vi "ChromaPowerSupply.vi"() -> ()   [LabVIEW 2018, in "Visualization.lvlib" / "VisualizeAcPwr.lvclass"]
doc: "This VI listens for any measurement data associated with the provided PluginName and displays it to the user for analysis. The display is only suitable for data coming from the RoomAlert Plugin."
uses:
  VisualizeAcPwr.lvclass
  VisualizeBase/VisualizeBase_class/SubVIs/VisualizationOptions.ctl
  <vilib>/Utility/miscctls.llb/LVRectTypeDef.ctl
  Loop Parameters.ctl
  AcPwr/AcPwrShared/clMeasurmentData.ctl
  AcPwr/AcPwrPlugins/AcPwrBaseClass/TypeDefs/SetParameterInputs.ctl
  AcPwr/AcPwrPlugins/ChromaPowerSupplyClass/TypeDefs/Device(s)Settings.ctl
  AcPwr/AcPwrPlugins/ChromaPowerSupplyClass/TypeDefs/Measurements.ctl
  <vilib>/event_ctls.llb/usereventprio.ctl
  VisualizeBase/VisualizeBase_class/Requests/VisUserEventType.ctl
  <vilib>/Utility/error.llb/Error Cluster From Error Code.vi
  <vilib>/ErrorRing/Error Ring.xnode
  <userlib>/NIST/NISTErrorLib/NISTErrorLib.lvlib
  VisualizeBase/VisualizeBase_class/VisualizeBase.lvclass
  TestClass/Test.lvclass
  Sensor/VisualizeSensor.lvclass
  StatusAndLog/VisualizeStatus.lvclass
  AcPwr/AcPwrShared/AcPwrShared.lvlib
  AcPwr/AcPwrPlugins/ChromaPowerSupplyClass/ChromaPowerSupply.lvclass
  AcPwr/AcPwrModule/AcPwrModule.lvlib
  AcPwr/AcPwrPlugins/AcPwrPlugins.lvlib
  AcPwr/AcPwrPlugins/AcPwrBaseClass/AcPwrBase.lvclass
panel:
  out "Writetime":u32 caption="Sample Write Time(ms)"
  out "ExitHelperLoops?":bool
  in  "Display":enum16{"Raw Data", "Voltage Vs Current"}(ring)
  in  "btnPause":bool
  out "VisualizationProperties":T1={"PauseAtStartup"=TRUE, "LogData"=FALSE, "LaunchInSubPanel"=TRUE, "FPMonitor"=0, "FPWindowBounds"={"Left"=0, "Top"=0, "Right"=0, "Bottom"=0}, "MonitorBounds"={"Left"=0, "Top"=0, "Right"=0, "Bottom"=0}, "MeasIndices"=[]}
  in  "INIFilePath":path
  in  "ModuleID":i32
  in  "Log Data":bool=TRUE
  in  "btnStop":bool
  in  "btnReset":bool
  in  "btnClearTest":bool
  in  "btnStopModule":bool
  out "XY Graph":cluster{dbl[], dbl[]}(graph)
  out "Chart":waveform(dbl)[](graph)=[{"t0"=timestamp(3657200531.6397257 s since 1904-01-01), "dt"=1.0, "Y"=[46.19]}, {"t0"=timestamp(3657200531.6397257 s since 1904-01-01), "dt"=1.0, "Y"=[2.0]}, {"t0"=timestamp(3657200531.6397257 s since 1904-01-01), "dt"=1.0, "Y"=[60.0]}]
  in  "Current":bool
  in  "Voltage":bool
  in  "Current (A)":dbl
  in  "Voltage (V)":dbl
  in  "btnStopParameterLoop":bool
  in  "btnRunParamLoop":bool
  in  "Loop Parameters":T3={"Parameter"=enum."Voltage", "Start Value"=5.0, "Increment"=1.0, "Interval (s)"=3.0, "# Iterations"=6, "End Value"=10.0} {"# Iterations" min=1; "Increment" format="%#.4f"}
  out "ErrorArray":errorcluster[](array[cluster])
  out "Incorrect DataType?":bool
  out "String Results":string
  in  "PluginName":string="Sensor.RoomAlert1"
  # "Set Parameter"
  # "Parameter Looping"
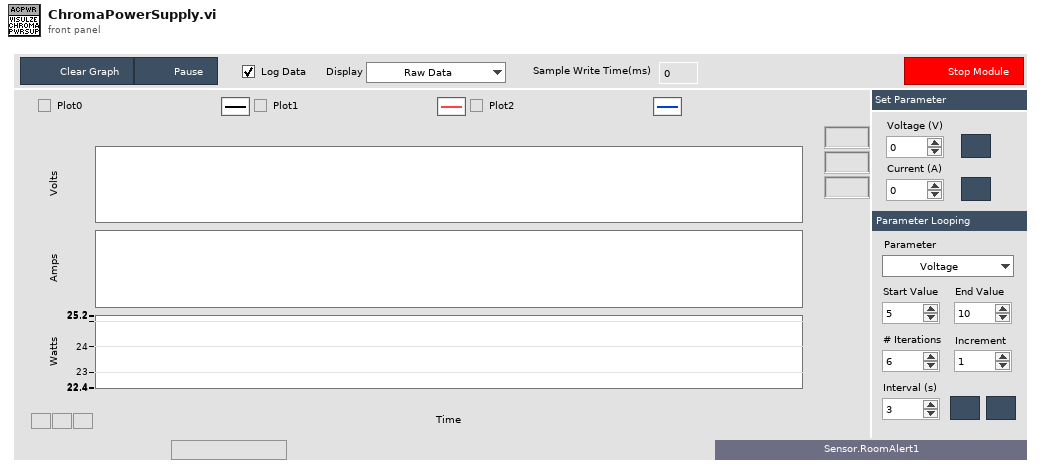
[diagram p1: front panel]
types:
  T1 = typedef "Visualization.lvlib/VisualizeBase.lvclass/VisualizationOptions.ctl" = cluster{"PauseAtStartup":bool, "LogData":bool, "LaunchInSubPanel":bool, "FPMonitor":u16, "FPWindowBounds":T2, "MonitorBounds":cluster{"Left":i16, "Top":i16, "Right":i16, "Bottom":i16}, "MeasIndices":i32[]}
  T2 = typedef "LVRectTypeDef.ctl" = cluster{"Left":i16, "Top":i16, "Right":i16, "Bottom":i16}
  T3 = typedef "Loop Parameters.ctl" = cluster{"Parameter":enum16{"Voltage", "Current", "Power", "Resistance"}, "Start Value":dbl, "Increment":dbl, "Interval (s)":dbl, "# Iterations":u32, "End Value":dbl}
  T4 = enum16{"open", "open or create", "create or replace", "create", "open (read-only)"}
  T5 = typedef "Visualization.lvlib/VisualizeBase.lvclass/VisRequestEvents.ctl" = cluster{"StopRequest":refnum<user-event>, "ResetRequest":refnum<user-event>, "FP Pop In or Out":refnum<user-event>}
  T6 = typedef "AcPwrShared.lvlib/AcPwrBroadcastEvents.ctl" = cluster{"DidInit":refnum<user-event>, "StatusUpdate":refnum<user-event>, "ErrorReport":refnum<user-event>, "DidStop":refnum<user-event>, "PathToINI":refnum<user-event>, "Measurements":refnum<user-event>, "LoadConfigFile":refnum<user-event>, "GetSettings":refnum<user-event>, "SetSettings":refnum<user-event>, "GetType&ID":refnum<user-event>, "GotSettings":refnum<user-event>, "GotSettingsLV":refnum<user-event>, "ParameterSet":refnum<user-event>}
  T7 = typedef "Visualization.lvlib/VisualizeBase.lvclass/VisFrmWrkBroadcastEvents.ctl" = cluster{"StatusUpdate":refnum<user-event>, "DidStop":refnum<user-event>, "NewModuleLoaded":refnum<user-event>, "StopVisualization":refnum<user-event>}
  T8 = typedef "AcPwrShared.lvlib/clMeasurmentData.ctl" = cluster{"MeasName":string, "XML Data":string, "WaveformData":waveform(dbl)[]}
  T9 = typedef "AcPwrPlugins.lvlib/AcPwrBase.lvclass/SetParameterInputs.ctl" = cluster{"Type":string, "Parameter":string, "Phase":i32, "Value":dbl, "Command":string, "Time Stamp":timestamp}
  T10 = typedef "AcPwrPlugins.lvlib/ChromaPowerSupply.lvclass/Device(s)Settings.ctl" = cluster{"Phases":cluster{"Handle":string, "Instrument Options":string, "id query (T)":bool, "reset device (T)":bool, "Timing":cluster{"TimingOn":enum16{""}, "Hours":u32, "Minutes":u32, "Seconds":dbl, "CutoffVoltage":dbl}, "Connected":bool, "Output Mode":enum16{"Voltage (DC)", "Current (DC)"}, "Voltage":dbl, "Current":dbl, "High Voltage Limit":dbl, "High Current Limit":dbl, "Power Protect":dbl, "Current Protect":dbl, "Voltage Protect":dbl, "Low Current Limit":dbl, "Low Voltage Limit":dbl, "Current Slew Rate":dbl, "Voltage Slew Rate":dbl, "Current Slew Infinite?":bool}[], "MeasName":string}
  T11 = typedef "AcPwrPlugins.lvlib/ChromaPowerSupply.lvclass/Measurements.ctl" = cluster{"Handle":string, "Name":string, "Enabled":bool, "Measurement Value":dbl, "btnMeasFetch":bool, "ProtectionStatusString":string, "Measurement Type":enum16{"Voltage", "Current", "Power"}}[]
  T12 = cluster{"Device Settings":T10, "Measurements":T11}
  T13 = typedef "Visualization.lvlib/VisualizeBase.lvclass/VisUserEventType.ctl" = cluster{"BusIndex":i8, "Data":variant}
  T14 = typedef "usereventprio.ctl" = enum32{"high priority", "normal priority"}
  T15 = cluster{"Handle":string, "Instrument Options":string, "id query (T)":bool, "reset device (T)":bool, "Timing":cluster{"TimingOn":enum16{""}, "Hours":u32, "Minutes":u32, "Seconds":dbl, "CutoffVoltage":dbl}, "Connected":bool, "Output Mode":enum16{"Voltage (DC)", "Current (DC)"}, "Voltage":dbl, "Current":dbl, "High Voltage Limit":dbl, "High Current Limit":dbl, "Power Protect":dbl, "Current Protect":dbl, "Voltage Protect":dbl, "Low Current Limit":dbl, "Low Voltage Limit":dbl, "Current Slew Rate":dbl, "Voltage Slew Rate":dbl, "Current Slew Infinite?":bool}[]
  T16 = cluster{"Handle":string, "Instrument Options":string, "id query (T)":bool, "reset device (T)":bool, "Timing":cluster{"TimingOn":enum16{""}, "Hours":u32, "Minutes":u32, "Seconds":dbl, "CutoffVoltage":dbl}, "Connected":bool, "Output Mode":enum16{"Voltage (DC)", "Current (DC)"}, "Voltage":dbl, "Current":dbl, "High Voltage Limit":dbl, "High Current Limit":dbl, "Power Protect":dbl, "Current Protect":dbl, "Voltage Protect":dbl, "Low Current Limit":dbl, "Low Voltage Limit":dbl, "Current Slew Rate":dbl, "Voltage Slew Rate":dbl, "Current Slew Infinite?":bool}
  T17 = typedef "sizeaction.ctl" = enum32{"Minimized", "Maximized", "Resized"}
  T18 = enum16{"Voltage", "Current", "Power", "Resistance"}
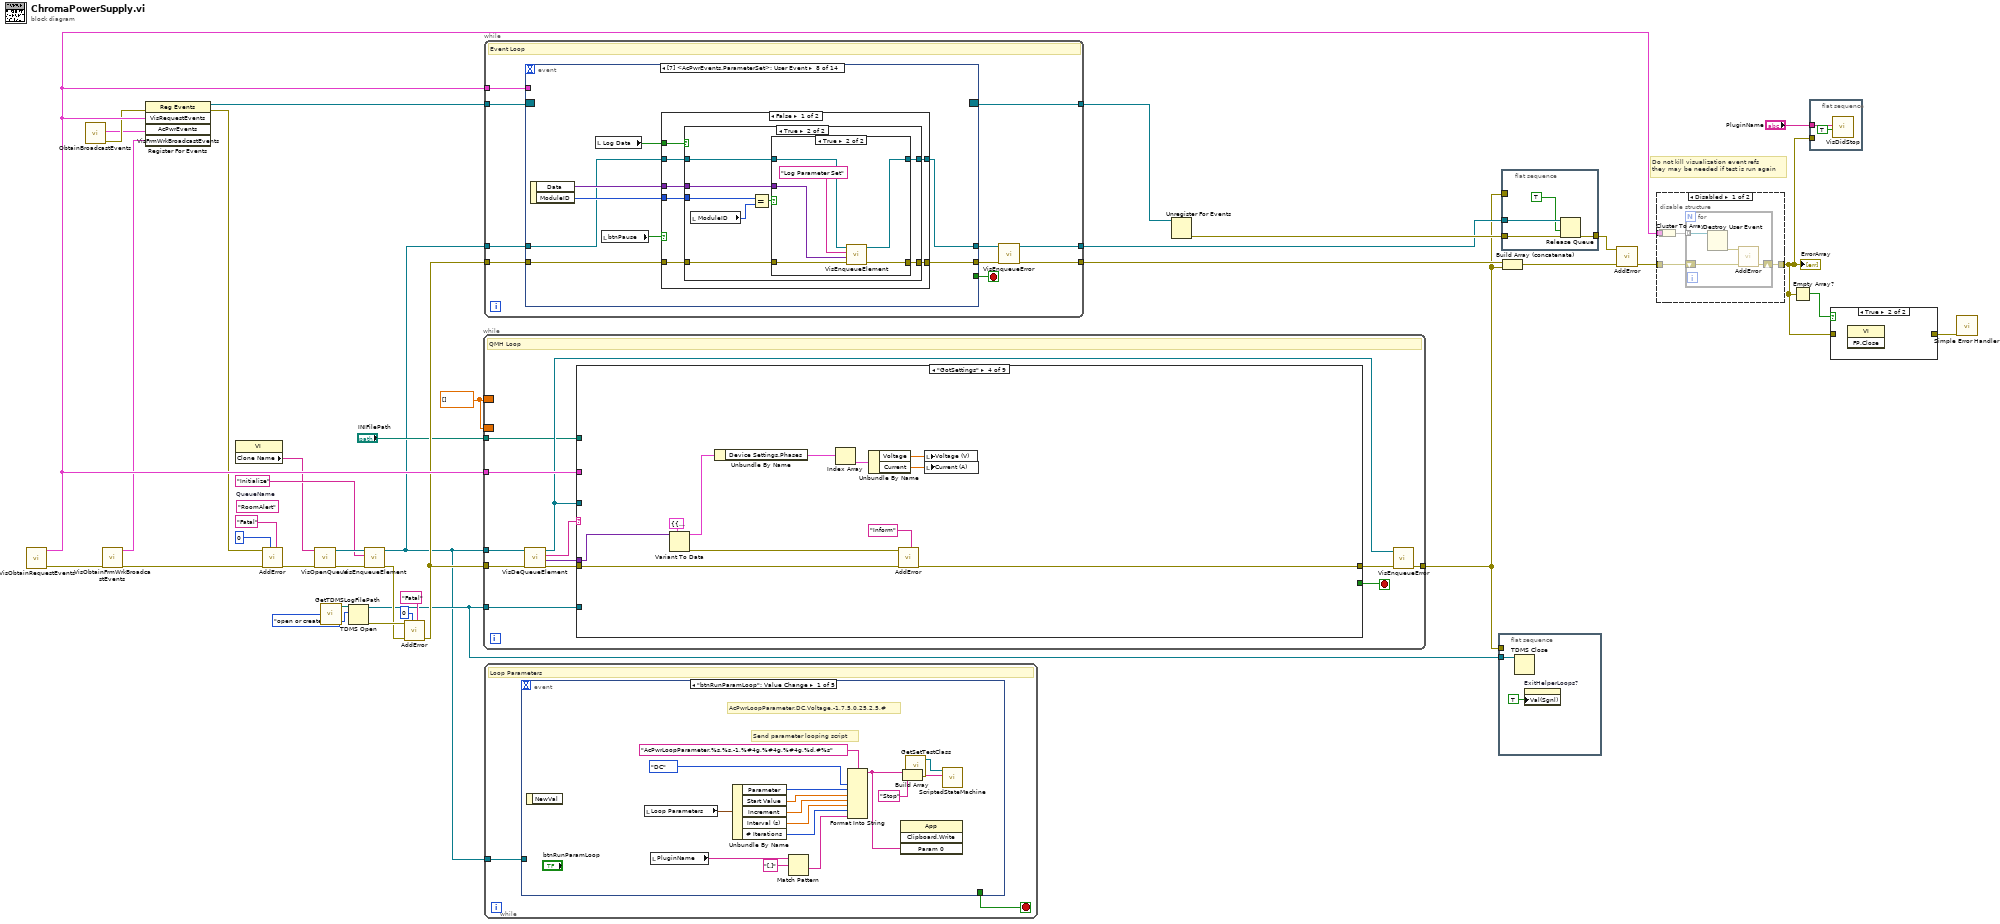
[diagram p0: block diagram]
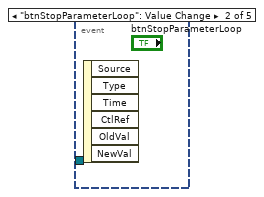
[diagram p2: hidden frame]
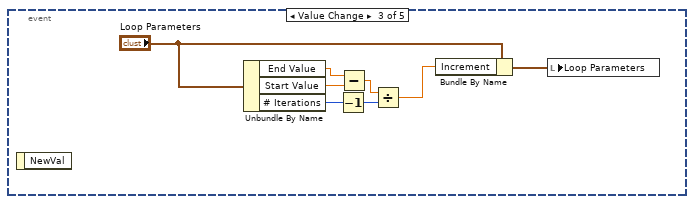
[diagram p3: hidden frame]
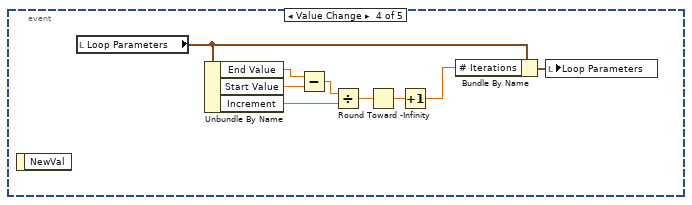
[diagram p4: hidden frame]
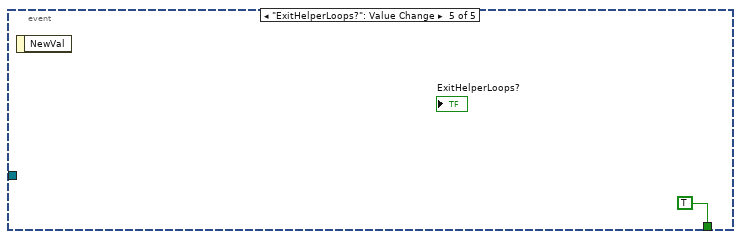
[diagram p5: hidden frame]
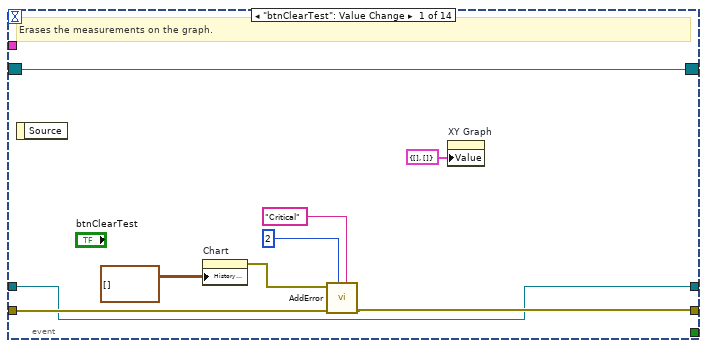
[diagram p7: hidden frame]
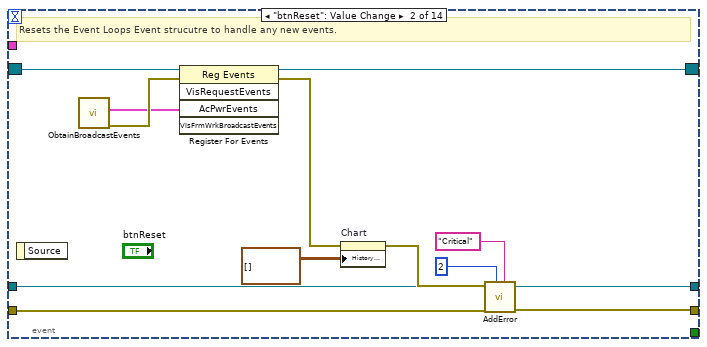
[diagram p8: hidden frame]
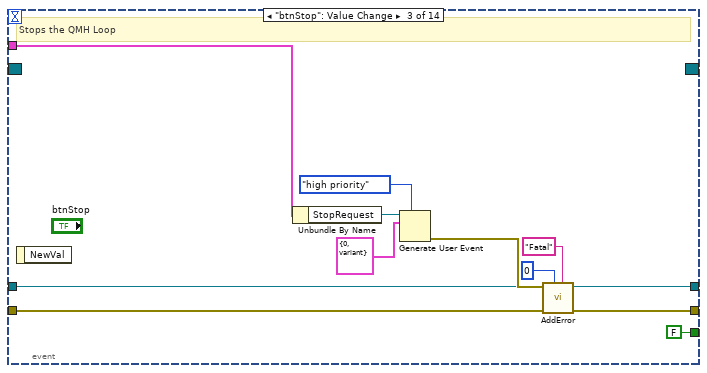
[diagram p9: hidden frame]
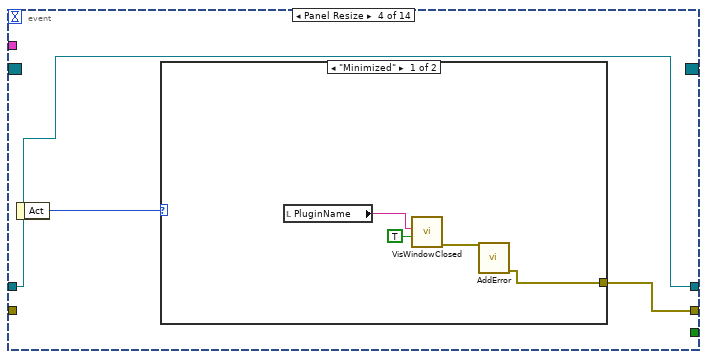
[diagram p10: hidden frame]
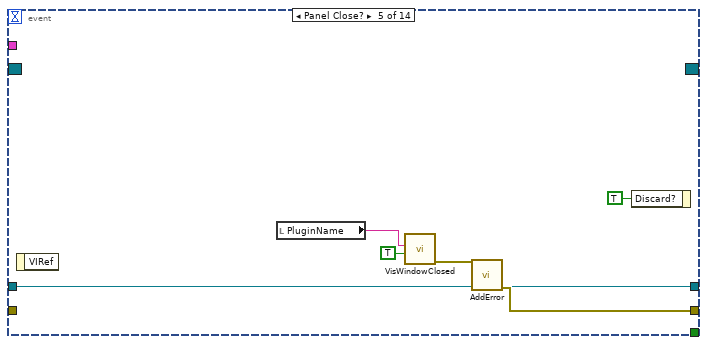
[diagram p12: hidden frame]
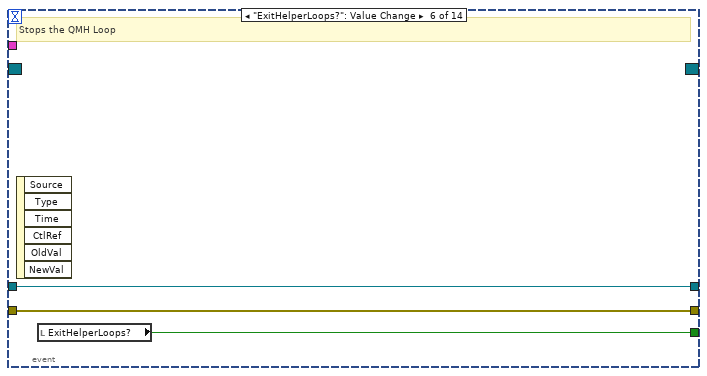
[diagram p13: hidden frame]
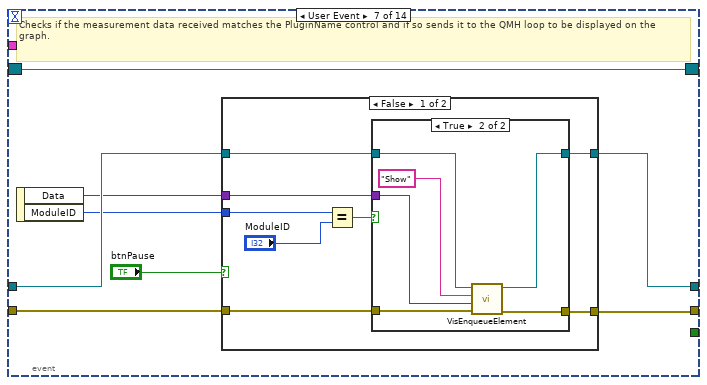
[diagram p14: hidden frame]
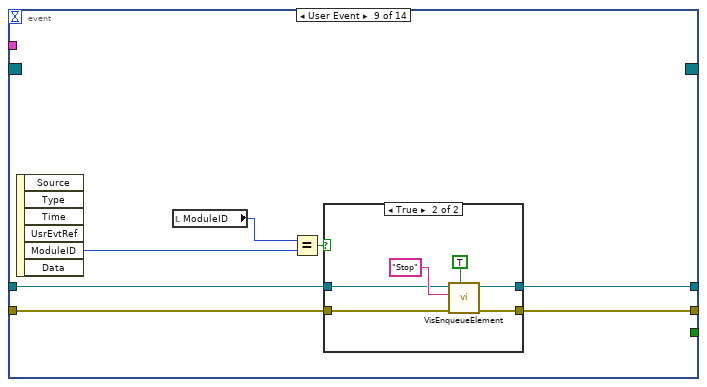
[diagram p20: hidden frame]
diagram:
  w1 = dbl[] []
  (unwired) "RoomAlert"  # QueueName
  # "Do not kill visualization event refs\nthey may be needed if test is run again"
  n1 = call "VisObtainRequestEvents.vi"() -> ("Error"=w29:errorcluster[], "VisRequestEvents"=w31:T5)  [unwired: 10 in]
  n2 = call "ObtainBroadcastEvents.vi"() -> ("error out"=w25:errorcluster, "AcPwrEvents"=w18:T6)  [unwired: 10 in]
  n3 = call "VisObtainFrmWrkBroadcastEvents.vi"("Error"=w29) -> ("Error"=w4:errorcluster[], "VisFrmWrkBroadcastEvents"=w3:T7)  [unwired: 9 in]
  n4 = register-events(error in=w25, w31, w18, w3) -> (reference out=w38:refnum<event-registration>, error out=w28:errorcluster)  [unwired: 1 in]
  n5 = property class="VI"() -> ("Clone Name"=w17:string)  [unwired: 2 in, 2 out]
  n6 = call <userlib>:"AddError.vi"("Severity"="Fatal", "Priority"=u8 0, "ErrorArray In"=w4, "error in (no error)"=w28) -> ("ErrorArray Out"=w24:errorcluster[])  [unwired: 6 in, 1 out]
  n7 = call "VisOpenQueue.vi"("Error Array In"=w24, "QueueName"=w17) -> ("Error Array Out"=w22:errorcluster[], "queue out"=w23:refnum<queue>)  [unwired: 8 in]
  n8 = call "GetTDMSLogFilePath.vi"() -> ("TDMS Log File Path"=w16:path)  [unwired: 11 in]
  n9 = TDMS Open(10:T4."open or create" ("operation (0:open)"), 11:w16) -> (0:w13:errorcluster, 3:w9:refnum<k34>)  [unwired: 5 in]
  n10 = call "VisEnqueueElement.vi"("Error Array In"=w22, "Message"="Initialize", "queue in"=w23) -> ("Error Array Out"=w12:errorcluster[], "queue out"=w2:refnum<queue>)  [unwired: 7 in]
  n11 = call <userlib>:"AddError.vi"("Severity"="Fatal", "Priority"=u8 0, "ErrorArray In"=w12, "error in (no error)"=w13) -> ("ErrorArray Out"=w11:errorcluster[])  [unwired: 6 in, 1 out]
  n12 = while {
    tunnel: w11 -> [w44]
    tunnel: [w47] -> w8
    tunnel: w2 -> [w43]
    tunnel: w31 -> [w49]
    tunnel: w9 -> [w40]
    tunnel: "INIFilePath" -> [w39]
    border: w1 -> [_]
    border: w1 -> [_]
    stop <- w50 stop-if-true
    # "QMH Loop"
    n13 = call "VisDeQueueElement.vi"("Error Array In"=w44, "Queue In"=w43) -> ("Error Array Out"=w42:errorcluster[], "Data"=w45:variant, "Message"=w46:string, "Queue Out"=w41:refnum<queue>)  [unwired: 6 in]
    n14 = case shown="\"GotSettings\"" w46 {
      selector: w46 -> [_ _ _ _ w174 _ _ _ _]
      tunnel: w45 -> [_ w72 w139 w164 _ w193 _ _ w235]
      tunnel: w42 -> [w61 w73 _ w162 w172 _ w222 _ w230]
      tunnel: [w54 w74 _ w161 w171 w183 w221 _ w232] -> w48
      tunnel: [_ _ _ _ _ w189 TRUE _ _] -> w50
      tunnel: w49 -> [_ _ _ _ _ w188 _ _ _]
      tunnel: w41 -> [_ _ _ _ _ w187 _ _ _]
      tunnel: w40 -> [_ w71 w138 _ _ _ _ _ _]
      tunnel: w39 -> [w60 _ _ _ _ _ w223 _ _]
      frame "Initialize" {
        n15 = property on="Chart" class="WFChart (strict)"("History Data"=waveform(dbl)[][] []) -> ()  [unwired: 2 in, 2 out]
        n16 = property on="XY Graph" class="XYGraph (strict)"("Value"=cluster{dbl[], dbl[]} {[], []} ("XY Graph")) -> ()  [unwired: 2 in, 2 out]
        n17 = call "ApplyVisOptions.vi"("INIFilePath"=w60) -> ("error out"=w64:errorcluster, "VisualizationProperties"=→"VisualizationProperties":T1)  [unwired: 9 in]
        n18 = call <userlib>:"AddError.vi"("Severity"="Inform", "ErrorArray In"=w61, "error in (no error)"=w64) -> ("ErrorArray Out"=w62:errorcluster[])  [unwired: 7 in, 1 out]
        n19 = property on="Display" class="Enum (strict)"("Val(Sgnl)"="Display") -> ()  [unwired: 2 in, 2 out]
        n20 = local read "ModuleID"() -> (w51:i32)
        n21 = call "GetSettingsRequestLV.vi"("SettingsToGet"=variant, "ModuleID"=w51) -> ("Error Out"=w53:errorcluster)  [unwired: 9 in]
        n22 = call <userlib>:"AddError.vi"("Severity"="Inform", "ErrorArray In"=w62, "error in (no error)"=w53) -> ("ErrorArray Out"=w54:errorcluster[])  [unwired: 7 in, 1 out]
      }
      frame "Show" {
        n23 = flat-sequence {
          tunnel: w71 -> [w76]
          tunnel: w72 -> [w77]
          tunnel: w73 -> [w78]
          tunnel: [w78] -> w70
          tunnel: [w77] -> w69
          tunnel: [w76] -> w68
          tunnel: [w75] -> w67
          tunnel: w70 -> [w92]
          tunnel: w69 -> [w91]
          tunnel: w68 -> [w86]
          tunnel: w67 -> [w79]
          tunnel: [w93] -> w66
          tunnel: [w79] -> w65
          tunnel: [w136] -> w74
          tunnel: w66 -> [w136]
          tunnel: w65 -> [w134]
          frame #0 {
            n24 = Tick Count (ms)() -> (millisecond timer value=w75:u32)
          }
          frame #1 {
            w88 = u32[] [0, 1, 2]  # PlotYAxis
            # "0=Left Axis and 1=Right Axis"
            n25 = Variant To Data(type=T8 {"MeasName"="", "XML Data"="", "WaveformData"=[]} ("MeasurmentDataCluster"), Variant=w91) -> (data=w89:T8, error out=w90:errorcluster)  [unwired: 1 in]
            n26 = control-ref of="Chart"() -> (w80:refnum<vi>)
            n27 = Unbundle By Name(w89) -> ("WaveformData"=w81:waveform(dbl)[])
            n28 = call "RetrieveAcPwrMeasurementData.vi"("WaveformChartReference"=w80, "PlotYScale"=w88, "WaveformArrayIn"=w81, "error in (no error)"=w90) -> ("WaveformArrayOut"=w83:waveform(dbl)[], "OutputString(Chroma)"=w85:string, "Incorrect DataType?"=w84:bool, "error out"=w87:errorcluster)  [unwired: 7 in, 1 out]
            n29 = case shown="False" w84 {
              selector: w84 -> [w107 _]
              tunnel: [w116 w132] -> w93
              tunnel: w92 -> [w115 w132]
              tunnel: w87 -> [w112 _]
              tunnel: w86 -> [w109 _]
              tunnel: w85 -> [w108 _]
              tunnel: w83 -> [w95 _]
              frame False {
                n30 = Array Size(array=w95) -> (size(s)=w94:i32)
                n31 = Index Array(array=w95, index #1=1 ("index"), index #2=0 ("index")) -> (element #1=w106:waveform(dbl), element #2=w105:waveform(dbl))
                n32 = property on="Chart" class="WFChart (strict)"("LegNumRows"=w94) -> ()  [unwired: 2 in, 2 out]
                n33 = Unbundle By Name(w106) -> ("Y"=w104:dbl[])
                n34 = Unbundle By Name(w105) -> ("Y"=w101:dbl[])
                n35 = feedback #1() -> (w103:dbl[])
                n36 = Build Array (concatenate)(w103, w104) -> (w98:dbl[])
                n37 = feedback-in #1(w98) -> ()
                n38 = feedback #2() -> (w102:dbl[])
                n39 = Build Array (concatenate)(w102, w101) -> (w97:dbl[])
                n40 = feedback-in #2(w97) -> ()
                n41 = Bundle(w98, w97) -> (→"XY Graph":cluster{dbl[], dbl[]})  [unwired: 1 in]
                n42 = case shown="True" "Log Data" {
                  tunnel: w112 -> [w117 w130]
                  tunnel: [w117 w131] -> w111
                  tunnel: w95 -> [_ w129]
                  tunnel: w109 -> [_ w124]
                  frame False {
                  }
                  frame True {
                    n43 = call "PrepareWaveformDataForTDMS.vi"("error in (no error)"=w130, "WaveformArray in"=w129) -> ("error out"=w128:errorcluster, "Measurement Data"=w126:dbl[][], "Channel Names"=w127:string[], "TimeStamp"=w119:timestamp)  [unwired: 6 in]
                    n44 = local read "PluginName"() -> (w122:string)
                    n45 = Build Array(w119) -> (w118:timestamp[])
                    n46 = TDMS Write(0:w124, 5:w122, 7:"TimeStamp" ("PluginName"), 9:w118, 11:w128) -> (4:w123:refnum<k34>, 6:w121:string, 15:w125:errorcluster)  [unwired: 1 in, 1 out]
                    n47 = TDMS Write(0:w123, 5:w121, 7:w127, 9:w126, 11:w125) -> (15:w131:errorcluster)  [unwired: 1 in, 3 out]
                  }
                }
                n48 = call <userlib>:"AddError.vi"("Severity"="Fatal" ("String"), "Priority"=u8 0, "ErrorArray In"=w115, "error in (no error)"=w111) -> ("ErrorArray Out"=w116:errorcluster[])  [unwired: 6 in, 1 out]
                "String Results" <- w108
                "Incorrect DataType?" <- w107
                "Chart" <- w95
              }
              frame True {
              }
            }
          }
          frame #2 {
            n49 = Tick Count (ms)() -> (millisecond timer value=w135:u32)
            n50 = Subtract(x=w135, y=w134) -> (x-y=→"Writetime":u32)
          }
        }
      }
      frame "Log Parameter Set" {
        n51 = Variant To Data(type=T9 {"Type"="", "Parameter"="", "Phase"=0, "Value"=0.0, "Command"="", "Time Stamp"=timestamp(0 s since 1904-01-01)}, Variant=w139) -> (data=w151:T9, error out=w140:errorcluster)  [unwired: 1 in]
        n52 = Unbundle By Name(w151) -> ("Type"=w150:string, "Parameter"=w149:string, "Phase"=w148:i32, "Time Stamp"=w144:timestamp, "Value"=w142:dbl)
        n53 = local read "PluginName"() -> (w137:string)
        n54 = Format Into String(format string="Set-%s_%s_Phase_%d", w150, w149, w148) -> (resulting string=w143:string)  [unwired: 2 in, 1 out]
        n55 = Concatenate Strings(w143, "_TimeStamp" ("string")) -> (w145:string)
        n56 = Build Array(w144) -> (w152:timestamp[])
        n57 = Build Array(w142) -> (w141:dbl[])
        n58 = TDMS Write(0:w138, 5:w137, 7:w145, 9:w152, 11:w140) -> (4:w154:refnum<k34>, 6:w153:string, 15:w155:errorcluster)  [unwired: 1 in, 1 out]
        n59 = TDMS Write(0:w154, 5:w153, 7:w143, 9:w141, 11:w155) -> ()  [unwired: 1 in, 4 out]
      }
      frame "GotSettings" {
        n60 = Variant To Data(type=T12 {"Device Settings"={"Phases"=[], "MeasName"=""}, "Measurements"=[]} ("output cluster"), Variant=w164) -> (data=w165:T12, error out=w160:errorcluster)  [unwired: 1 in]
        n61 = Unbundle By Name(w165) -> ("Device Settings.Phases"=w166:T15)
        n62 = Index Array(array=w166) -> (element=w167:T16)  [unwired: 1 in]
        n63 = Unbundle By Name(w167) -> ("Voltage"=w158:dbl, "Current"=w157:dbl)
        n64 = call <userlib>:"AddError.vi"("Severity"="Inform", "ErrorArray In"=w162, "error in (no error)"=w160) -> ("ErrorArray Out"=w161:errorcluster[])  [unwired: 7 in, 1 out]
        n65 = local write "Voltage (V)"(w158) -> ()
        n66 = local write "Current (A)"(w157) -> ()
      }
      frame Default {
        n67 = xnode "Error Ring"("parameter 0"=w174) -> ("error out"=w173:errorcluster)
        n68 = call <userlib>:"AddError.vi"("Severity"="Inform" ("String"), "Priority"=u8 5, "ErrorArray In"=w172, "error in (no error)"=w173) -> ("ErrorArray Out"=w171:errorcluster[], "error out"=w170:errorcluster)  [unwired: 6 in]
        n69 = call <vilib>:"Clear Errors.vi"("error in (no error)"=w170) -> ()  [unwired: 5 in, 2 out]
      }
      frame "Error" {
        n70 = Variant To Data(type=errorcluster[] [], Variant=w193) -> (data=w191:errorcluster[], error out=w182:errorcluster)  [unwired: 1 in]
        n71 = call <userlib>:"ParseErrors.vi"("ErrorArray"=w191) -> ("ErrorArray"=w190:errorcluster[])  [unwired: 8 in, 2 out]
        n72 = for {
          tunnel: w190 -> [w204] mode=indexing
          tunnel: [w198] -> w184 mode=concatenating
          tunnel: [w196] -> w189
          tunnel: w188 -> [w195]
          tunnel: w187 -> [w194]
          stop <- w196 stop-if-true
          n73 = call <userlib>:"GeneralHandler.vi"("error in (no error)"=w204) -> ("Severity"=w197:string, "Stop"=w201:bool, "Abort"=w202:bool, "Continue"=w203:bool)  [unwired: 6 in, 1 out]
          n74 = Build Array(w203, w202, w201) -> (w200:bool[])
          n75 = Boolean Array To Number(Boolean array=w200) -> (number=w199:u32)
          n76 = case shown="1" w199 {
            tunnel: [_ _ w209 w218] -> w198
            tunnel: w197 -> [_ _ _ w211]
            tunnel: [_ _ _ w213] -> w196
            tunnel: w195 -> [_ _ _ w212]
            tunnel: w194 -> [_ _ w205 _]
            frame 0, Default {
              # "No Dialog"
            }
            frame 1 {
              # "Continue"
            }
            frame 2 {
              # "Abort, Flush Queue"
              n77 = Flush Queue(queue=w205) -> (error out=w208:errorcluster)  [unwired: 1 in, 2 out]
              n78 = call <userlib>:"AddError.vi"("Severity"="Critical" ("String"), "Priority"=u8 1, "error in (no error)"=w208) -> ("ErrorArray Out"=w209:errorcluster[])  [unwired: 7 in, 1 out]
            }
            frame 4 {
              # "Stop"
              n79 = Unbundle By Name(w212) -> ("StopRequest"=w219:refnum<user-event>)
              n80 = Equal?(x=w211, y="Fatal" ("x")) -> (x = y?=w213:bool)
              n81 = Generate User Event(priority (normal)=usereventprio."high priority", user event=w219, event data cluster=T13 {"BusIndex"=0, "Data"=variant} ("event data")) -> (error out=w217:errorcluster)  [unwired: 1 in, 1 out]
              n82 = call <userlib>:"AddError.vi"("error in (no error)"=w217) -> ("ErrorArray Out"=w218:errorcluster[], "error out"=w214:errorcluster)  [unwired: 9 in]
              n83 = call <vilib>:"Clear Errors.vi"("error in (no error)"=w214) -> ()  [unwired: 5 in, 2 out]
            }
          }
        }
        n84 = call <userlib>:"AddError.vi"("Severity"="Critical", "Priority"=u8 2, "ErrorArray In"=w184, "error in (no error)"=w182) -> ("ErrorArray Out"=w183:errorcluster[])  [unwired: 6 in, 1 out]
      }
      frame "Stop" {
        n85 = local read "VisualizationProperties"() -> (w220:T1)
        n86 = call "WriteVisOptionsToINIFile.vi"("Visualization Options"=w220, "INIFilePath"=w223) -> ("error out"=w224:errorcluster)  [unwired: 8 in, 1 out]
        n87 = call <userlib>:"AddError.vi"("Severity"="Inform", "ErrorArray In"=w222, "error in (no error)"=w224) -> ("ErrorArray Out"=w221:errorcluster[])  [unwired: 7 in, 1 out]
      }
      frame "- ---AcPwr Module Specific Commands----" {
      }
      frame "Set Parameter" {
        n88 = Variant To Data(type="", Variant=w235) -> (data=w233:string, error out=w231:errorcluster)  [unwired: 1 in]
        n89 = call <userlib>:"AddError.vi"("Severity"="Inform", "Priority"=u8 0, "ErrorArray In"=w230, "error in (no error)"=w231) -> ("ErrorArray Out"=w227:errorcluster[])  [unwired: 6 in, 1 out]
        n90 = local read "PluginName"() -> (w243:string)
        n91 = case shown="\"False\", Default" w233 {
          tunnel: "Voltage (V)" -> [_ w254 _]
          tunnel: "Current (A)" -> [_ _ w255]
          tunnel: [_ w254 w255] -> w245
          tunnel: [TRUE _ _] -> w242
          frame "False", Default {
          }
          frame "Voltage" {
          }
          frame "Current" {
          }
        }
        n92 = Match Pattern(string=w243, regular expression="[.]") -> (after substring=w244:string)  [unwired: 1 in, 3 out]
        n93 = Format Into String(format string="AcPwrSetParameter,%s,%s,-1,%.4f,#%s", enum16{"AC", "DC"}."DC" ("input 1"), w233, w245, w244) -> (resulting string=w241:string)  [unwired: 2 in, 1 out]
        n94 = case shown="False" w242 {
          tunnel: w241 -> [w250 _]
          tunnel: [w248 w252] -> w232
          tunnel: w227 -> [w246 w252]
          frame False {
            n95 = call "GetSetTestClass.vi"() -> ("Test.lvclass"=w251:refnum<class "Test.lvclass">)  [unwired: 11 in]
            n96 = Build Array(w250, "Stop" ("element")) -> (w249:string[])
            n97 = call "ScriptedStateMachine.vi"("ErrorArray 2"=w246, "script"=w249, "Test.lvclass 2"=w251) -> ("ErrorArray"=w248:errorcluster[])  [unwired: 6 in, 2 out]
          }
          frame True {
          }
        }
      }
    }
    n98 = call "VisEnqueueError.vi"("Error Array In"=w48, "Queue in"=w41) -> ("Error Array Out"=w47:errorcluster[])  [unwired: 8 in, 1 out]
  }
  n99 = while {
    tunnel: w38 -> [w265]
    tunnel: [w259] -> w36
    tunnel: [w263] -> w37
    tunnel: w31 -> [w262]
    tunnel: w11 -> [w261]
    tunnel: w2 -> [w260]
    tunnel: [w256] -> w20
    stop <- w264 stop-if-true
    # "Event Loop"
    n100 = event shown="[7] <AcPwrEvents.ParameterSet>: User Event" {
      selector: w265 -> [w268 w286 _ _ _ _ w317 _ _ _ _ _ _ _]
      dyn-events: [w268 w285 _ _ _ _ w317 _ _ _ _ _ _ _] -> w263
      timeout: _ -> [_ _ _ _ _ _ _ _ _ _ _ _ _ _]
      tunnel: [_ _ FALSE ("Priority? (F)") _ _ w311 _ _ _ _ _ _ _ _] -> w264
      tunnel: [w271 w283 w290 w299 w306 w312 w319 w340 w378 _ w400 w408 w419 w429] -> w258
      tunnel: w262 -> [_ _ w289 _ _ _ _ _ _ _ _ _ _ _]
      tunnel: w261 -> [w272 w284 w297 _ _ w312 w320 w342 w377 _ _ w406 _ w428]
      tunnel: w260 -> [w266 w276 w287 w298 w305 w313 w321 w343 w380 w390 w398 w405 w418 w431]
      tunnel: [w266 w276 w287 w298 w305 w313 w318 w341 w379 w390 w399 w407 w418 w430] -> w257
      event "btnClearTest": Value Change {
        # "Erases the measurements on the graph."
        n101 = event-data() -> ()  [unwired: 1 in, 1 out]
        n102 = property on="Chart" class="WFChart (strict)"("History Data"=waveform(dbl)[][] []) -> (error out=w270:errorcluster)  [unwired: 2 in, 1 out]
        n103 = call <userlib>:"AddError.vi"("Severity"="Critical", "Priority"=u8 2, "ErrorArray In"=w272, "error in (no error)"=w270) -> ("ErrorArray Out"=w271:errorcluster[])  [unwired: 6 in, 1 out]
        n104 = property on="XY Graph" class="XYGraph (strict)"("Value"=cluster{dbl[], dbl[]} {[], []} ("XY Graph")) -> ()  [unwired: 2 in, 2 out]
      }
      event "btnReset": Value Change {
        # "Resets the Event Loops Event strucutre to handle any new events."
        n105 = event-data() -> ()  [unwired: 1 in, 1 out]
        n106 = call "ObtainBroadcastEvents.vi"() -> ("error out"=w277:errorcluster, "AcPwrEvents"=w275:T6)  [unwired: 10 in]
        n107 = register-events(reference=w286, error in=w277, w275) -> (reference out=w285:refnum<event-registration>, error out=w279:errorcluster)  [unwired: 2 in]
        n108 = property on="Chart" class="WFChart (strict)"(error in=w279, "History Data"=waveform(dbl)[][] []) -> (error out=w278:errorcluster)  [unwired: 1 in, 1 out]
        n109 = call <userlib>:"AddError.vi"("Severity"="Critical", "Priority"=u8 2, "ErrorArray In"=w284, "error in (no error)"=w278) -> ("ErrorArray Out"=w283:errorcluster[])  [unwired: 6 in, 1 out]
      }
      event "btnStop": Value Change {
        # "Stops the QMH Loop"
        n110 = event-data() -> ()  [unwired: 1 in, 1 out]
        n111 = Unbundle By Name(w289) -> ("StopRequest"=w295:refnum<user-event>)
        n112 = Generate User Event(priority (normal)=usereventprio."high priority", user event=w295, event data cluster=T13 {"BusIndex"=0, "Data"=variant} ("event data")) -> (error out=w296:errorcluster)  [unwired: 1 in, 1 out]
        n113 = call <userlib>:"AddError.vi"("Severity"="Fatal" ("String"), "Priority"=u8 0, "ErrorArray In"=w297, "error in (no error)"=w296) -> ("ErrorArray Out"=w290:errorcluster[])  [unwired: 6 in, 1 out]
      }
      event Panel Resize {
        n114 = event-data() -> ("Act"=w300:T17)  [unwired: 1 in]
        n115 = case shown="\"Minimized\"" w300 {
          tunnel: [w301 _] -> w299
          frame "Minimized" {
            n116 = local read "PluginName"() -> (w303:string)
            n117 = call "VisWindowClosed.vi"("Window Closed?"=TRUE ("Window Minimized or Clozed?"), "Module Name"=w303) -> ("error out"=w304:errorcluster)  [unwired: 9 in]
            n118 = call <userlib>:"AddError.vi"("error in (no error)"=w304) -> ("ErrorArray Out"=w301:errorcluster[])  [unwired: 9 in, 1 out]
          }
          frame "Maximized", Default {
          }
        }
      }
      event Panel Close? {
        n119 = event-data() -> ()  [unwired: 1 in, 1 out]
        n120 = local read "PluginName"() -> (w307:string)
        n121 = call "VisWindowClosed.vi"("Window Closed?"=TRUE ("Window Minimized or Clozed?"), "Module Name"=w307) -> ("error out"=w308:errorcluster)  [unwired: 9 in]
        n122 = call <userlib>:"AddError.vi"("error in (no error)"=w308) -> ("ErrorArray Out"=w306:errorcluster[])  [unwired: 9 in, 1 out]
        n123 = event-data("Discard?"=TRUE) -> ()  [unwired: 1 in, 1 out]
      }
      event "ExitHelperLoops?": Value Change {
        # "Stops the QMH Loop"
        n124 = event-data() -> ()  [unwired: 1 in, 6 out]
        n125 = local read "ExitHelperLoops?"() -> (w311:bool)
      }
      event User Event {
        # "Checks if the measurement data received matches the PluginName control and if so sends it to the QMH loop to be displayed on the graph."
        n126 = event-data() -> ("Data"=w316:variant, "ModuleID"=w315:i32)  [unwired: 1 in]
        n127 = case shown="False" "btnPause" {
          tunnel: w321 -> [w329 w339]
          tunnel: w320 -> [w328 w338]
          tunnel: [w327 w338] -> w319
          tunnel: [w326 w339] -> w318
          tunnel: w316 -> [w325 _]
          tunnel: w315 -> [w322 _]
          frame False {
            n128 = Equal?(x=w322, y="ModuleID") -> (x = y?=w324:bool)
            n129 = case shown="True" w324 {
              tunnel: [w330 w336] -> w327
              tunnel: w329 -> [w331 w335]
              tunnel: w328 -> [w330 w337]
              tunnel: [w331 w333] -> w326
              tunnel: w325 -> [_ w334]
              frame False {
              }
              frame True {
                n130 = call "VisEnqueueElement.vi"("Error Array In"=w337, "Data"=w334, "Message"="Show", "queue in"=w335) -> ("Error Array Out"=w336:errorcluster[], "queue out"=w333:refnum<queue>)  [unwired: 6 in]
              }
            }
          }
          frame True {
          }
        }
      }
      event User Event {
        n131 = event-data() -> ("Data"=w345:variant, "ModuleID"=w344:i32)  [unwired: 1 in]
        n132 = local read "Log Data"() -> (w346:bool)
        n133 = local read "btnPause"() -> (w347:bool)
        n134 = case shown="False" w347 {
          tunnel: w343 -> [w354 w374]
          tunnel: w342 -> [w353 w373]
          tunnel: [w352 w373] -> w340
          tunnel: [w351 w374] -> w341
          tunnel: w345 -> [w350 _]
          tunnel: w344 -> [w349 _]
          tunnel: w346 -> [w348 _]
          frame False {
            n135 = case shown="True" w348 {
              tunnel: w354 -> [w356 w364]
              tunnel: w353 -> [w355 w363]
              tunnel: [w355 w362] -> w352
              tunnel: [w356 w361] -> w351
              tunnel: w350 -> [_ w360]
              tunnel: w349 -> [_ w358]
              frame False {
              }
              frame True {
                n136 = local read "ModuleID"() -> (w357:i32)
                n137 = Equal?(x=w358, y=w357) -> (x = y?=w359:bool)
                n138 = case shown="True" w359 {
                  tunnel: [w365 w371] -> w362
                  tunnel: w364 -> [w366 w370]
                  tunnel: w363 -> [w365 w372]
                  tunnel: [w366 w368] -> w361
                  tunnel: w360 -> [_ w369]
                  frame False {
                  }
                  frame True {
                    n139 = call "VisEnqueueElement.vi"("Error Array In"=w372, "Data"=w369, "Message"="Log Parameter Set", "queue in"=w370) -> ("Error Array Out"=w371:errorcluster[], "queue out"=w368:refnum<queue>)  [unwired: 6 in]
                  }
                }
              }
            }
          }
          frame True {
          }
        }
      }
      event User Event {
        n140 = event-data() -> ("ModuleID"=w376:i32)  [unwired: 1 in, 5 out]
        n141 = local read "ModuleID"() -> (w375:i32)
        n142 = Equal?(x=w375, y=w376) -> (x = y?=w381:bool)
        n143 = case shown="True" w381 {
          tunnel: [w382 w387] -> w378
          tunnel: [w383 w386] -> w379
          tunnel: w380 -> [w383 w385]
          tunnel: w377 -> [w382 w384]
          frame False {
          }
          frame True {
            n144 = call "VisEnqueueElement.vi"("Priority? (F)"=TRUE, "Error Array In"=w384, "Message"="Stop", "queue in"=w385) -> ("Error Array Out"=w387:errorcluster[], "queue out"=w386:refnum<queue>)  [unwired: 6 in]
          }
        }
      }
      event "Display": Value Change {
        n145 = event-data() -> ("NewVal"=w393:enum16{"Raw Data", "Voltage Vs Current"})  [unwired: 1 in]
        n146 = case shown="\"Raw Data\", Default" w393 {
          tunnel: [TRUE FALSE] -> w392
          frame "Raw Data", Default {
          }
          frame "Voltage Vs Current" {
          }
        }
        n147 = Not(x=w392) -> (.not. x?=w391:bool)
        n148 = property on="Chart" class="WFChart (strict)"("Visible"=w392) -> ()  [unwired: 2 in, 2 out]
        n149 = property on="XY Graph" class="XYGraph (strict)"("Visible"=w391) -> ()  [unwired: 2 in, 2 out]
      }
      event "Voltage", "Current": Value Change {
        n150 = event-data() -> ("CtlRef"=w401:refnum<vi>)  [unwired: 1 in]
        n151 = property class="Bool"(reference=w401) -> ("Label.Text"=w396:string)  [unwired: 1 in, 2 out]
        n152 = call "VisEnqueueElement.vi"("Data"=w396, "Message"="Set Parameter", "queue in"=w398) -> ("Error Array Out"=w400:errorcluster[], "queue out"=w399:refnum<queue>)  [unwired: 7 in]
      }
      event User Event {
        n153 = event-data() -> ("ModuleID"=w403:i32, "Data"=w402:variant)  [unwired: 1 in]
        n154 = local read "ModuleID"() -> (w404:i32)
        n155 = Equal?(x=w404, y=w403) -> (x = y?=w409:bool)
        n156 = case shown="True" w409 {
          tunnel: w405 -> [w410 w416]
          tunnel: w406 -> [w411 w415]
          tunnel: [w410 w414] -> w407
          tunnel: [w411 w413] -> w408
          tunnel: w402 -> [_ w412]
          frame False {
          }
          frame True {
            (unwired) TRUE ("Priority? (F)")
            n157 = call "VisEnqueueElement.vi"("Error Array In"=w415, "Data"=w412, "Message"="GotSettings", "queue in"=w416) -> ("Error Array Out"=w413:errorcluster[], "queue out"=w414:refnum<queue>)  [unwired: 6 in]
          }
        }
      }
      event "btnStopModule": Value Change {
        n158 = event-data() -> ()  [unwired: 1 in, 1 out]
        n159 = local read "ModuleID"() -> (w421:i32)
        n160 = call "StatusUpdateByModID.vi"("Status"="User requested module stop", "Accessors:Module ID"=w421) -> ("error out"=w422:errorcluster)  [unwired: 9 in]
        n161 = flat-sequence {
          tunnel: [w424] -> w419
          tunnel: w422 -> [_]
          frame #0 {
            n162 = local read "PluginName"() -> (w423:string)
            n163 = call "GetSetTestClass.vi"() -> ("Test.lvclass"=w425:refnum<class "Test.lvclass">)  [unwired: 11 in]
            n164 = call "StopModByName.vi"("Module Name"=w423, "Test.lvclass"=w425) -> ("ErrorArray Out"=w424:errorcluster[])  [unwired: 4 in, 5 out]
          }
        }
      }
      event User Event {
        # "Framework requested visualization stop"
        n165 = event-data() -> ("Data"=w426:variant)  [unwired: 1 in]
        n166 = local read "PluginName"() -> (w427:string)
        n167 = Variant To Data(type="" ("Message"), Variant=w426) -> (data=w437:string, error out=w435:errorcluster)  [unwired: 1 in]
        n168 = call <userlib>:"AddError.vi"("Severity"="Inform", "Priority"=u8 3, "ErrorArray In"=w428, "error in (no error)"=w435) -> ("ErrorArray Out"=w434:errorcluster[])  [unwired: 6 in, 1 out]
        n169 = Equal?(x=w427, y=w437) -> (x = y?=w436:bool)
        n170 = case shown="True" w436 {
          tunnel: w431 -> [w440 w444]
          tunnel: [w439 w443] -> w429
          tunnel: w434 -> [w439 w442]
          tunnel: [w440 w441] -> w430
          frame False {
          }
          frame True {
            n171 = call "VisEnqueueElement.vi"("Priority? (F)"=TRUE, "Error Array In"=w442, "Message"="Stop", "queue in"=w444) -> ("Error Array Out"=w443:errorcluster[], "queue out"=w441:refnum<queue>)  [unwired: 6 in]
          }
        }
      }
    }
    n172 = call "VisEnqueueError.vi"("Error Array In"=w258, "Queue in"=w257) -> ("Error Array Out"=w259:errorcluster[], "Queue out"=w256:refnum<queue>)  [unwired: 8 in]
  }
  n173 = while {
    tunnel: w2 -> [w447]
    stop <- w448 stop-if-true
    # "Loop Parameters"
    n174 = event shown="[0] \"btnRunParamLoop\": Value Change" {
      selector: _ -> [_ _ _ _ _]
      dyn-events: _ -> [_ _ _ _ _]
      timeout: _ -> [_ _ _ _ _]
      tunnel: [_ _ _ _ TRUE] -> w448
      tunnel: w447 -> [_ _ _ _ _]
      event "btnRunParamLoop": Value Change {
        # "AcPwrLoopParameter,DC,Voltage,-1,7.5,0.25,2,5,#"
        # "Send parameter looping script"
        n175 = event-data() -> ()  [unwired: 1 in, 1 out]
        n176 = local read "Loop Parameters"() -> (w451:T3)
        n177 = local read "PluginName"() -> (w450:string)
        n178 = Unbundle By Name(w451) -> ("Parameter"=w462:T18, "Start Value"=w461:dbl, "Increment"=w460:dbl, "Interval (s)"=w459:dbl, "# Iterations"=w458:u32)
        n179 = Match Pattern(string=w450, regular expression="[.]") -> (after substring=w453:string)  [unwired: 1 in, 3 out]
        n180 = Format Into String(format string="AcPwrLoopParameter,%s,%s,-1,%#4g,%#4g,%#4g,%d,#%s", enum16{"AC", "DC"}."DC" ("input 1"), w462, w461, w460, w459, w458, w453) -> (resulting string=w449:string)  [unwired: 2 in, 1 out]
        n181 = invoke class="App" method="Clipboard.Write"("Param 0"=w449) -> ()  [unwired: 3 in, 4 out]
        n182 = Build Array(w449, "Stop" ("element")) -> (w455:string[])
        n183 = call "GetSetTestClass.vi"() -> ("Test.lvclass"=w454:refnum<class "Test.lvclass">)  [unwired: 11 in]
        n184 = call "ScriptedStateMachine.vi"("script"=w455, "Test.lvclass 2"=w454) -> ()  [unwired: 7 in, 3 out]
      }
      event "btnStopParameterLoop": Value Change {
        n185 = event-data() -> ()  [unwired: 1 in, 6 out]
      }
      event Value Change {
        n186 = event-data() -> ()  [unwired: 1 in, 1 out]
        n187 = Unbundle By Name("Loop Parameters") -> ("End Value"=w471:dbl, "Start Value"=w470:dbl, "# Iterations"=w468:u32)
        n188 = Decrement(x=w468) -> (x-1=w465:u32)
        n189 = Subtract(x=w471, y=w470) -> (x-y=w469:dbl)
        n190 = Divide(x=w469, y=w465) -> (x/y=w467:dbl)
        n191 = Bundle By Name(cluster="Loop Parameters", "Increment"=w467) -> (w466:T3)
        n192 = local write "Loop Parameters"(w466) -> ()
      }
      event Value Change {
        n193 = event-data() -> ()  [unwired: 1 in, 1 out]
        n194 = local read "Loop Parameters"() -> (w477:T3)
        n195 = Unbundle By Name(w477) -> ("End Value"=w480:dbl, "Start Value"=w479:dbl, "Increment"=w474:dbl)
        n196 = Subtract(x=w480, y=w479) -> (x-y=w478:dbl)
        n197 = Divide(x=w478, y=w474) -> (x/y=w476:dbl)
        n198 = Round Toward -Infinity(1:w476) -> (0:w473:dbl)
        n199 = Increment(x=w473) -> (x+1=w472:dbl)
        n200 = Bundle By Name(cluster=w477, "# Iterations"=w472) -> (w475:T3)
        n201 = local write "Loop Parameters"(w475) -> ()
      }
      event "ExitHelperLoops?": Value Change {
        n202 = event-data() -> ()  [unwired: 1 in, 1 out]
      }
    }
  }
  n203 = Unregister For Events(event registration refnum=w37) -> (error out=w35:errorcluster)  [unwired: 1 in]
  n204 = flat-sequence {
    tunnel: w9 -> [w483]
    tunnel: w8 -> [_]
    frame #0 {
      n205 = TDMS Close(11:w483) -> ()  [unwired: 1 in, 2 out]
      n206 = property on="ExitHelperLoops?" class="Bool (strict)"("Val(Sgnl)"=TRUE ("Value (Signaling)")) -> ()  [unwired: 2 in, 2 out]
    }
  }
  n207 = flat-sequence {
    tunnel: w35 -> [w487]
    tunnel: [w486] -> w33
    tunnel: w20 -> [w485]
    tunnel: w8 -> [_]
    frame #0 {
      n208 = Release Queue(queue=w485, force destroy? (F)=TRUE, error in (no error)=w487) -> (error out=w486:errorcluster)  [unwired: 2 out]
    }
  }
  n209 = Build Array (concatenate)(w36, w8) -> (w34:errorcluster[])
  n210 = call <userlib>:"AddError.vi"("ErrorArray In"=w34, "error in (no error)"=w33) -> ("ErrorArray Out"=w32:errorcluster[])  [unwired: 8 in, 1 out]
  n211 = disable-structure shown="Disabled" {
    disable-tunnel: w32 -> [w490 w496]
    disable-tunnel: w31 -> [w489 _]
    disable-tunnel: [w488 w496] -> w5
    frame Disabled {
      n212 = Cluster To Array(cluster=w489) -> (array=w491:refnum<user-event>[])
      n213 = for {
        tunnel: w491 -> [w495] mode=indexing
        shift-right: [w494] -> w488
        shift-left: w490 -> [w493]
        n214 = Destroy User Event(user event=w495) -> (error out=w492:errorcluster)  [unwired: 1 in]
        n215 = call <userlib>:"AddError.vi"("ErrorArray In"=w493, "error in (no error)"=w492) -> ("ErrorArray Out"=w494:errorcluster[])  [unwired: 8 in, 1 out]
      }
    }
    frame Enabled {
    }
  }
  "ErrorArray" <- w5
  n216 = Empty Array?(array=w5) -> (empty?=w30:bool)
  n217 = flat-sequence {
    tunnel: "PluginName" -> [w498]
    tunnel: w5 -> [_]
    frame #0 {
      n218 = call "VisDidStop.vi"("DidStop?"=TRUE, "Module Name"=w498) -> ()  [unwired: 9 in, 1 out]
    }
  }
  n219 = case shown="True" w30 {
    tunnel: [w499 _] -> w19
    tunnel: w5 -> [w500 _]
    frame False {
      n220 = Merge Errors(w500) -> (w499:errorcluster)
    }
    frame True {
      n221 = invoke class="VI" method="FP.Close"() -> ()  [unwired: 3 in, 3 out]
    }
  }
  n222 = call <vilib>:"Simple Error Handler.vi"("error in (no error)"=w19) -> ()  [unwired: 4 in, 5 out]
